vi "UpdateMetricCache.vi"(8 "error in (no error)":errorcluster, 9 "Metrics":variant, 11 "MetricDefinitionInstances":T2[](array[typedef])) -> (0 "error out":errorcluster, 1 "Metrics out":variant)   [LabVIEW 2015]
uses:
  <vilib>/addons/InsightCM/MessageBus/Base/controls/MetricDefinitionInstance.ctl
  <vilib>/addons/InsightCM/MessageBus/Base/controls/KeyValuePair.ctl
  <vilib>/addons/InsightCM/MessageBus/Base/controls/MetricChannelType.ctl
  <vilib>/addons/InsightCM/Utilities/Analysis/Shared/controls/BandDomain.ctl
  <vilib>/addons/InsightCM/Utilities/Analysis/Shared/controls/BandCalculation.ctl
  <vilib>/addons/InsightCM/Utilities/Analysis/Shared/AnalysisHelper.lvlib
panel:
  out "properties out":T1[](array[typedef])
  out "Properties":T1[](array[typedef])
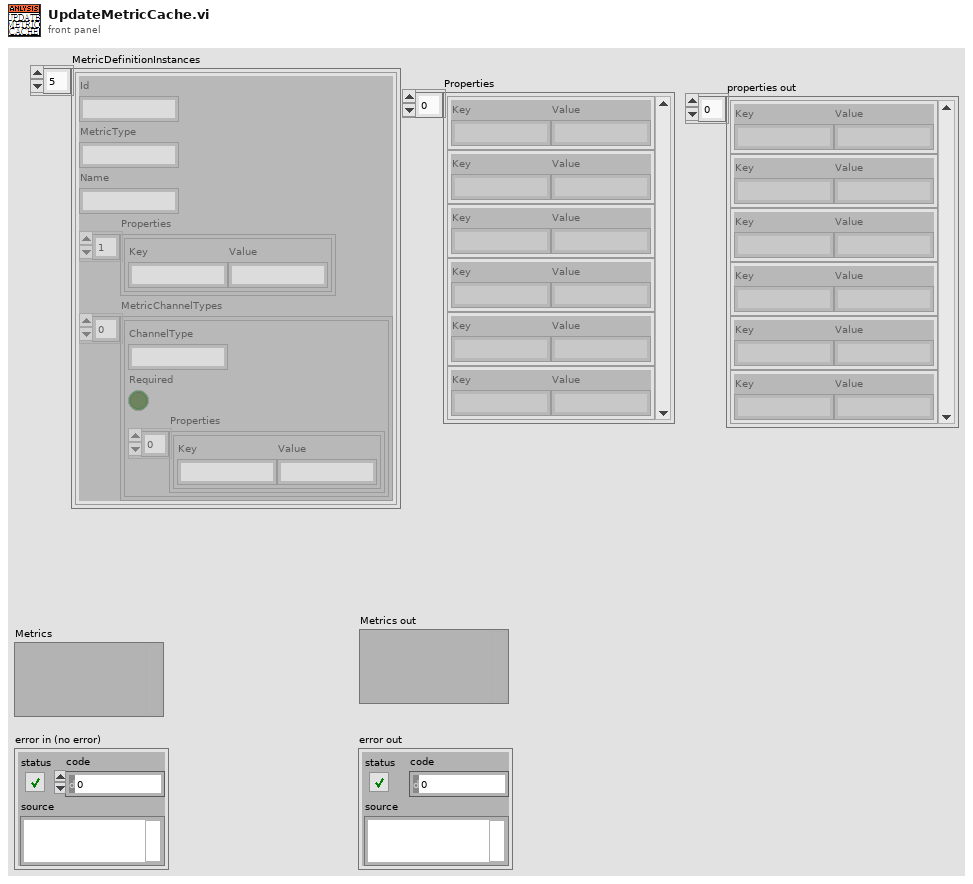
[diagram p1: front panel]
types:
  T1 = typedef "KeyValuePair.ctl" = cluster{"Key":string, "Value":string}
  T2 = typedef "MetricDefinitionInstance.ctl" = cluster{"Id":string, "MetricType":string, "Name":string, "Properties":T1[], "MetricChannelTypes":T3[]}
  T3 = typedef "MetricChannelType.ctl" = cluster{"ChannelType":string, "Required":bool, "Properties":T1[]}
  T4 = typedef "AnalysisHelper.lvlib/BandDomain.ctl" = enum16{"Frequency", "CPM", "Orders"}
  T5 = typedef "AnalysisHelper.lvlib/BandCalculation.ctl" = enum16{"Total", "Max", "Phase"}
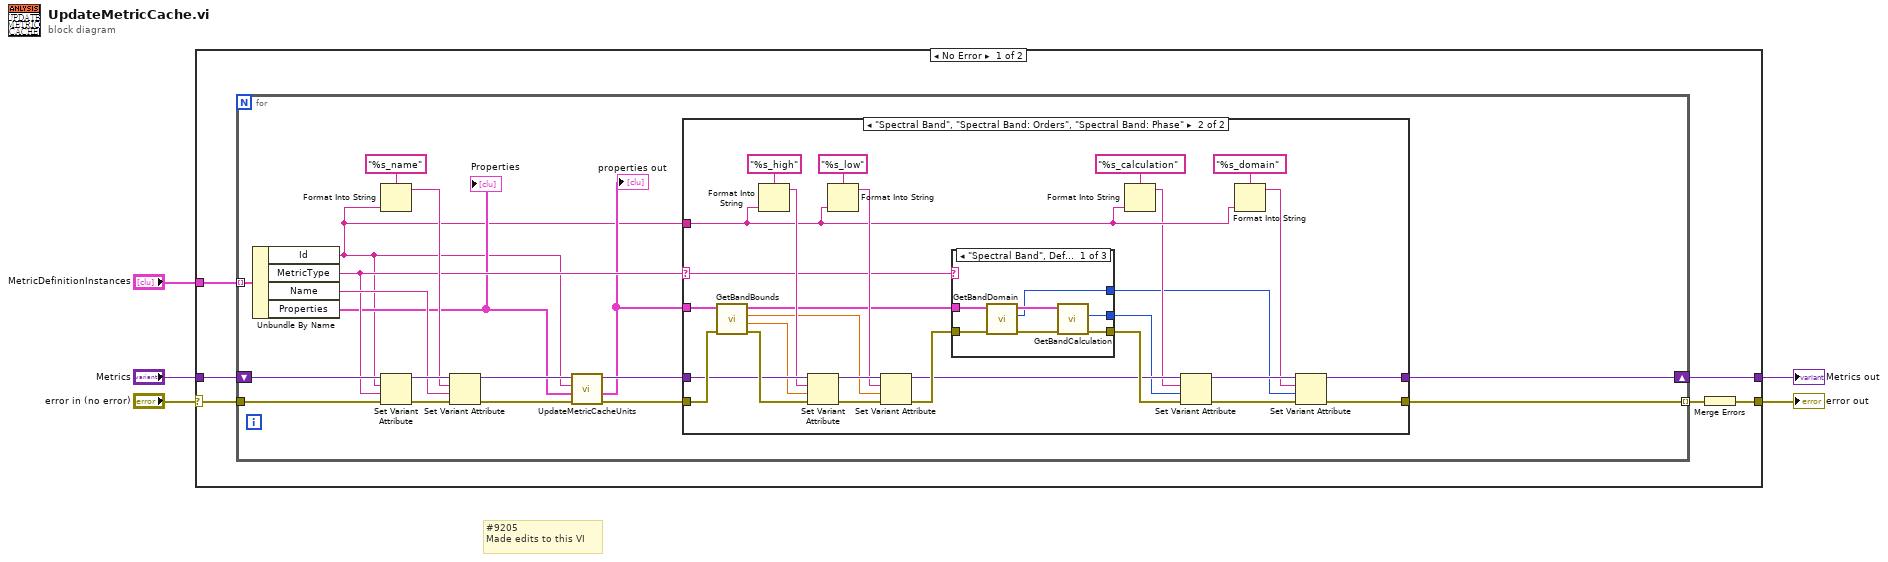
[diagram p0: block diagram]
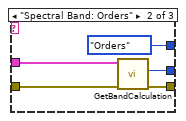
[diagram p3: hidden frame]
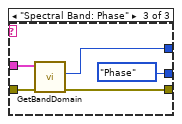
[diagram p4: hidden frame]
diagram:
  # "#9205\nMade edits to this VI"
  n1 = case shown="No Error" "error in (no error)" {
    selector: "error in (no error)" -> [w6 w78]
    tunnel: [w11 w78] -> w5
    tunnel: [w10 w77] -> w4
    tunnel: "Metrics" -> [w9 w77]
    tunnel: "MetricDefinitionInstances" -> [w7 _]
    frame No Error {
      n2 = for {
        tunnel: w7 -> [w29] mode=indexing
        tunnel: w6 -> [w28]
        shift-right: [w25] -> w10
        shift-left: w9 -> [w27]
        tunnel: [w26] -> w8 mode=indexing
        n3 = Unbundle By Name(w29) -> ("Id"=w12:string, "MetricType"=w19:string, "Name"=w20:string, "Properties"=w15:T1[])
        "Properties" <- w15
        n4 = Format Into String(format string="%s_name", w12) -> (resulting string=w21:string)  [unwired: 2 in, 1 out]
        n5 = Set Variant Attribute(Variant=w27, name=w12, value=w19, error in=w28) -> (Variant out=w23:variant, error out=w24:errorcluster)  [unwired: 1 out]
        n6 = Set Variant Attribute(Variant=w23, name=w21, value=w20, error in=w24) -> (Variant out=w17:variant, error out=w18:errorcluster)  [unwired: 1 out]
        n7 = call <vilib>:"UpdateMetricCacheUnits.vi"("error in (no error)"=w18, "properties"=w15, "metric definition instance id"=w12, "metric cache in"=w17) -> ("error out"=w14:errorcluster, "properties out"=w13:T1[], "metric cache out"=w16:variant)  [unwired: 5 in]
        "properties out" <- w13
        n8 = case shown="\"Spectral Band\", \"Spectral Band: Orders\", \"Spectral Band: Phase\"" w19 {
          selector: w19 -> [_ w46]
          tunnel: [w30 w39] -> w26
          tunnel: w14 -> [w30 w57]
          tunnel: [w31 w38] -> w25
          tunnel: w16 -> [w31 w55]
          tunnel: w13 -> [_ w59]
          tunnel: w12 -> [_ w42]
          frame Default {
          }
          frame "Spectral Band", "Spectral Band: Orders", "Spectral Band: Phase" {
            n9 = call "GetBandBounds.vi"("error in (no error)"=w57, "Properties In"=w59) -> ("error out"=w56:errorcluster, "High"=w53:sgl, "Low"=w48:sgl, "Properties Out"=w45:T1[])  [unwired: 6 in]
            n10 = Format Into String(format string="%s_high", w42) -> (resulting string=w50:string)  [unwired: 2 in, 1 out]
            n11 = Set Variant Attribute(Variant=w55, name=w50, value=w53, error in=w56) -> (Variant out=w54:variant, error out=w58:errorcluster)  [unwired: 1 out]
            n12 = Format Into String(format string="%s_low", w42) -> (resulting string=w49:string)  [unwired: 2 in, 1 out]
            n13 = Set Variant Attribute(Variant=w54, name=w49, value=w48, error in=w58) -> (Variant out=w36:variant, error out=w47:errorcluster)  [unwired: 1 out]
            n14 = case shown="\"Spectral Band\", Default" w46 {
              tunnel: w47 -> [w66 w68 w75]
              tunnel: w45 -> [w65 w69 w73]
              tunnel: [w62 w71 w74] -> w41
              tunnel: [w61 w70 BandCalculation."Phase" ("Calculation")] -> w35
              tunnel: [w60 BandDomain."Orders" ("Domain") w72] -> w33
              frame "Spectral Band", Default {
                n15 = call <vilib>:"GetBandDomain.vi"("error in (no error)"=w66, "Properties In"=w65) -> ("error out"=w63:errorcluster, "Domain"=w60:T4, "Properties Out"=w64:T1[])  [unwired: 7 in]
                n16 = call <vilib>:"GetBandCalculation.vi"("error in (no error)"=w63, "Properties In"=w64) -> ("error out"=w62:errorcluster, "Calculation"=w61:T5)  [unwired: 7 in, 1 out]
              }
              frame "Spectral Band: Orders" {
                n17 = call <vilib>:"GetBandCalculation.vi"("error in (no error)"=w68, "Properties In"=w69) -> ("error out"=w71:errorcluster, "Calculation"=w70:T5)  [unwired: 7 in, 1 out]
              }
              frame "Spectral Band: Phase" {
                n18 = call <vilib>:"GetBandDomain.vi"("error in (no error)"=w75, "Properties In"=w73) -> ("error out"=w74:errorcluster, "Domain"=w72:T4)  [unwired: 7 in, 1 out]
              }
            }
            n19 = Format Into String(format string="%s_calculation", w42) -> (resulting string=w34:string)  [unwired: 2 in, 1 out]
            n20 = Set Variant Attribute(Variant=w36, name=w34, value=w35, error in=w41) -> (Variant out=w37:variant, error out=w40:errorcluster)  [unwired: 1 out]
            n21 = Format Into String(format string="%s_domain", w42) -> (resulting string=w32:string)  [unwired: 2 in, 1 out]
            n22 = Set Variant Attribute(Variant=w37, name=w32, value=w33, error in=w40) -> (Variant out=w38:variant, error out=w39:errorcluster)  [unwired: 1 out]
          }
        }
      }
      n23 = Merge Errors(w8) -> (w11:errorcluster)
    }
    frame Error {
    }
  }
  "error out" <- w5
  "Metrics out" <- w4
